vi "GOLPI full test.vi"() -> ()   [LabVIEW 2013]
uses:
  Set Variable/Set - Scalar - Real.vi
  Get Variable/Get - Scalar - Real.vi
  Set Variable/Set - Scalar - Complex.vi
  Get Variable/Get - Scalar - Complex.vi
  Set Variable/Set - Matrix - Real.vi
  Get Variable/Get - Matrix - Reals.vi
  GOLPI library.lvlib
panel:
  out "result":bool[](array[boolean])
  out "GNU Octave version":string
  out "exit code":i32
  out "error out":errorcluster
  in  "Octave binary directory":path=path "C:/Program Files/Octave-3.6.2/bin"
  in  "Working directory":path=path "C:/"
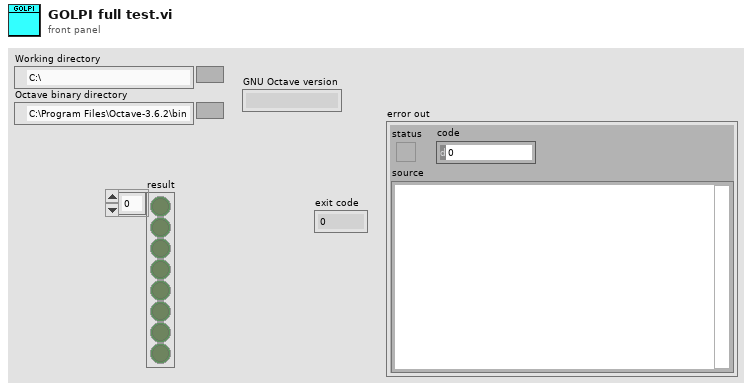
[diagram p1: front panel]
types:
  T1 = typedef "LV Process.lvlibp/Pipe Handle.ctl" = cluster{"lv_proc.dll file path":path, "process instance handle":u32[]}
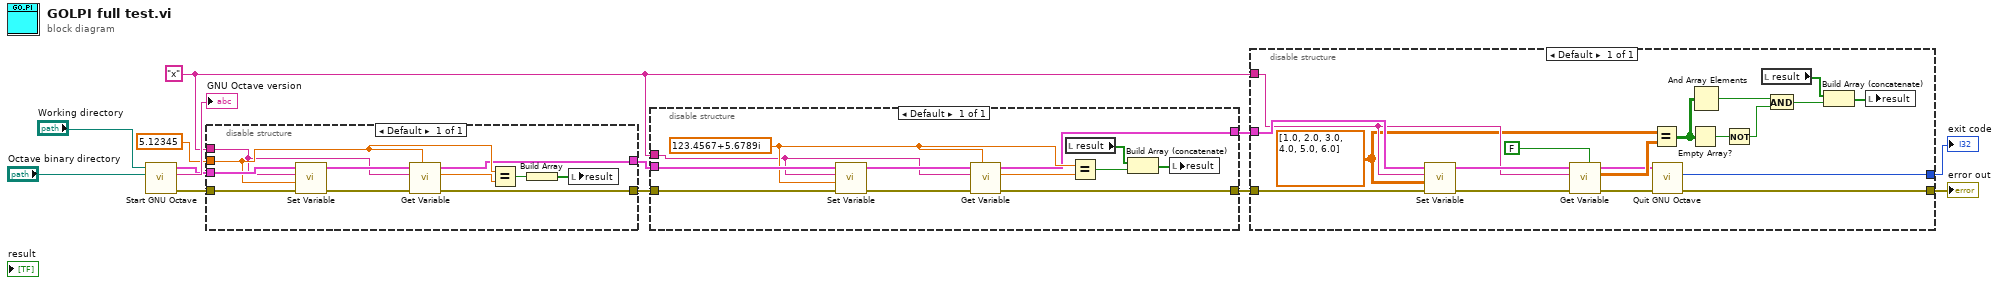
[diagram p0: block diagram]
diagram:
  w1 = "x" ("variable name")
  n1 = call "Start GNU Octave.vi"("Octave binary directory"="Octave binary directory", "Working directory"="Working directory") -> ("error out"=w8:errorcluster, "GNU Octave version"=→"GNU Octave version":string, "pipe out"=w7:T1)  [unwired: 6 in, 1 out]
  n2 = disable-structure shown="Default" {
    disable-tunnel: w8 -> [w23]
    disable-tunnel: w7 -> [w22]
    disable-tunnel: 5.12345 ("value") -> [w19]
    disable-tunnel: [w18] -> w5
    disable-tunnel: [w17] -> w4
    disable-tunnel: w1 -> [w16]
    frame Enabled {
      n3 = call-poly "Set Variable.vi"("error in"=w23, "value"=w19, "variable name"=w16, "pipe in"=w22) -> ("error out"=w21:errorcluster, "pipe out"=w20:T1)  [unwired: 6 in]
      n4 = call-poly "Get Variable.vi"("data type of variable"=w19, "error in"=w21, "variable name"=w16, "pipe in"=w20) -> ("error out"=w18:errorcluster, "value"=w24:dbl, "pipe out"=w17:T1)  [unwired: 5 in]
      n5 = Equal?(x=w19, y=w24) -> (x = y?=w15:bool)
      n6 = Build Array(w15) -> (w14:bool[])
      n7 = local write "result"(w14) -> ()
    }
  }
  n8 = disable-structure shown="Default" {
    disable-tunnel: w5 -> [w34]
    disable-tunnel: w4 -> [w33]
    disable-tunnel: [w30] -> w3
    disable-tunnel: [w29] -> w2
    disable-tunnel: w1 -> [w28]
    frame Enabled {
      w32 = cdb 123.4567+5.6789i ("value")
      n9 = call-poly "Set Variable.vi"("error in"=w34, "value"=w32, "variable name"=w28, "pipe in"=w33) -> ("error out"=w35:errorcluster, "pipe out"=w36:T1)  [unwired: 6 in]
      n10 = call-poly "Get Variable.vi"("data type of variable"=w32, "error in"=w35, "variable name"=w28, "pipe in"=w36) -> ("error out"=w29:errorcluster, "value"=w31:cdb, "pipe out"=w30:T1)  [unwired: 5 in]
      n11 = local read "result"() -> (w26:bool[])
      n12 = Equal?(x=w32, y=w31) -> (x = y?=w25:bool)
      n13 = Build Array (concatenate)(w26, w25) -> (w27:bool[])
      n14 = local write "result"(w27) -> ()
    }
  }
  n15 = disable-structure shown="Default" {
    disable-tunnel: [w55] -> w11
    disable-tunnel: [w54] -> w10
    disable-tunnel: w3 -> [w53]
    disable-tunnel: w2 -> [w52]
    disable-tunnel: w1 -> [w49]
    frame Enabled {
      w48 = dbl[][] [[1.0, 2.0, 3.0], [4.0, 5.0, 6.0]] ("value")
      n16 = call-poly "Set Variable.vi"("error in"=w52, "value"=w48, "variable name"=w49, "pipe in"=w53) -> ("error out"=w51:errorcluster, "pipe out"=w50:T1)  [unwired: 6 in]
      n17 = call-poly "Get Variable.vi"("use temporary file?"=FALSE, "error in"=w51, "variable name"=w49, "pipe in"=w50) -> ("error out"=w45:errorcluster, "value"=w47:dbl[][], "pipe out"=w46:T1)  [unwired: 5 in]
      n18 = Equal?(x=w48, y=w47) -> (x = y?=w41:bool[][])
      n19 = call "Quit GNU Octave.vi"("error in"=w45, "pipe in"=w46) -> ("error out"=w55:errorcluster, "exit code"=w54:i32)  [unwired: 8 in]
      n20 = Empty Array?(array=w41) -> (empty?=w40:bool)
      n21 = And Array Elements(Boolean array=w41) -> (logical AND=w38:bool)
      n22 = Not(x=w40) -> (.not. x?=w39:bool)
      n23 = local read "result"() -> (w43:bool[])
      n24 = And(x=w38, y=w39) -> (x .and. y?=w37:bool)
      n25 = Build Array (concatenate)(w43, w37) -> (w42:bool[])
      n26 = local write "result"(w42) -> ()
    }
  }
  "error out" <- w11
  "exit code" <- w10
